vi "Get Reference Out Frequency.vi"(8 "error in (no error)":errorcluster, 11 "Handle in":i32) -> (0 "error out":errorcluster, 2 "Reference out Frequency (Hz)":i32, 3 "Handle out":i32)   [LabVIEW 2013, in "Thorlabs_MC2000B.lvlib"]
doc: "Get actual frequency of blade spinning"
uses:
  <instrlib>/Thorlabs_MC2000B/Thorlabs_MC2000B.lvlib
  <instrlib>/Thorlabs_MC2000B/Library/MC2000CommandLibWin64.dll
  <instrlib>/Thorlabs_MC2000B/Library/MC2000CommandLibWin32.dll
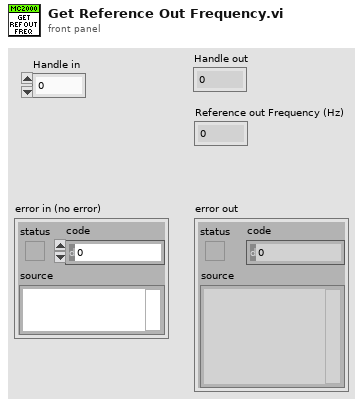
[diagram p1: front panel]
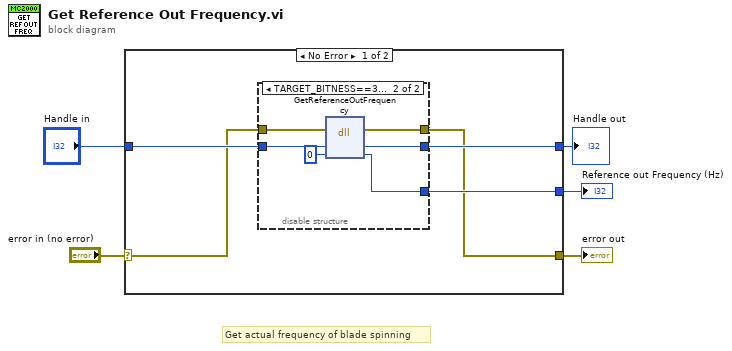
[diagram p0: block diagram]
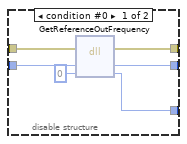
[diagram p2: hidden frame]
diagram:
  # "Get actual frequency of blade spinning"
  n1 = case shown="No Error" "error in (no error)" {
    selector: "error in (no error)" -> [w7 w24]
    tunnel: [w8 _] -> w5
    tunnel: [w6 w24] -> w4
    tunnel: "Handle in" -> [w10 w23]
    tunnel: [w9 w23] -> w1
    frame No Error {
      n2 = disable-structure shown="TARGET_BITNESS==32" {
        disable-tunnel: w10 -> [w16 w22]
        disable-tunnel: [w15 w21] -> w9
        disable-tunnel: [w14 w20] -> w8
        disable-tunnel: w7 -> [w12 w18]
        disable-tunnel: [w11 w17] -> w6
        frame condition #0 {
          n3 = dll-call lib="D:/Program Files/National Instruments/LabVIEW 2011/instr.lib/Thorlabs_MC2000B/Library/MC2000CommandLibWin64.dll" fn="GetReferenceOutFrequency"(error in=w12, "hdl"=w16, "freq"=0 ("input")) -> (error out=w11:errorcluster, "hdl"=w15:i32, "freq"=w14:i32)  [unwired: 3 in, 1 out]
        }
        frame condition #1 (active) {
          n4 = dll-call lib="C:/Program Files (x86)/National Instruments/LabVIEW 2013/instr.lib/Thorlabs_MC2000B/Library/MC2000CommandLibWin32.dll" fn="GetReferenceOutFrequency"(error in=w18, "hdl"=w22, "freq"=0 ("input")) -> (error out=w17:errorcluster, "hdl"=w21:i32, "freq"=w20:i32)  [unwired: 3 in, 1 out]
        }
      }
    }
    frame Error {
    }
  }
  "error out" <- w4
  "Reference out Frequency (Hz)" <- w5
  "Handle out" <- w1
